vi "Load-deposition-file.vi"(8 "error in (no error)":errorcluster, 11 "Object ref in":T1) -> (0 "error out":errorcluster, 1 "Succes?":bool, 3 "Object ref out":T1)   [LabVIEW 2013, in "SLMControl.lvlib" / "SC-Main.lvclass"]
uses:
  SC-Main.lvclass
  Object-reference.ctl
  Client/Sources/Supported-modules.ctl
  SC-Main.lvclass/SC-Main.ctl
  Read Deposition status.vi
  Read Deposition file index.vi
  Read Deposition files.vi
  Read Client.vi
  Client/Sources/SC-Client.lvclass
  SA-SLMAPI/Sources/Load-file/Load-file.lvclass
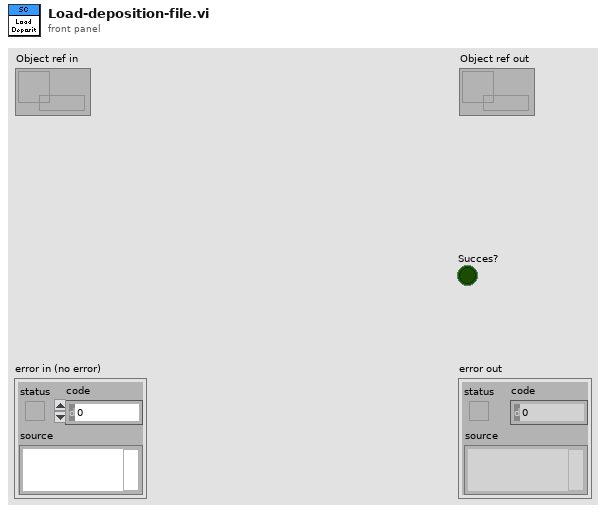
[diagram p1: front panel]
types:
  T1 = typedef "SLMControl.lvlib/SC-Main.lvclass/Object-reference.ctl" = refnum<data-value>
  T2 = typedef "SLMControl.lvlib/SC-Client.lvclass/Supported-modules.ctl" = enum16{"Server", "All", "SLMControl", "PowderDeposition", "StrategyParser", "CameraVision", "MaterialCharacterization", "StatusMonitor", "SLMSimulation", "LaserCharacterization"}
  T3 = typedef "SLMControl.lvlib/SC-Client.lvclass/Object-reference.ctl" = refnum<data-value>
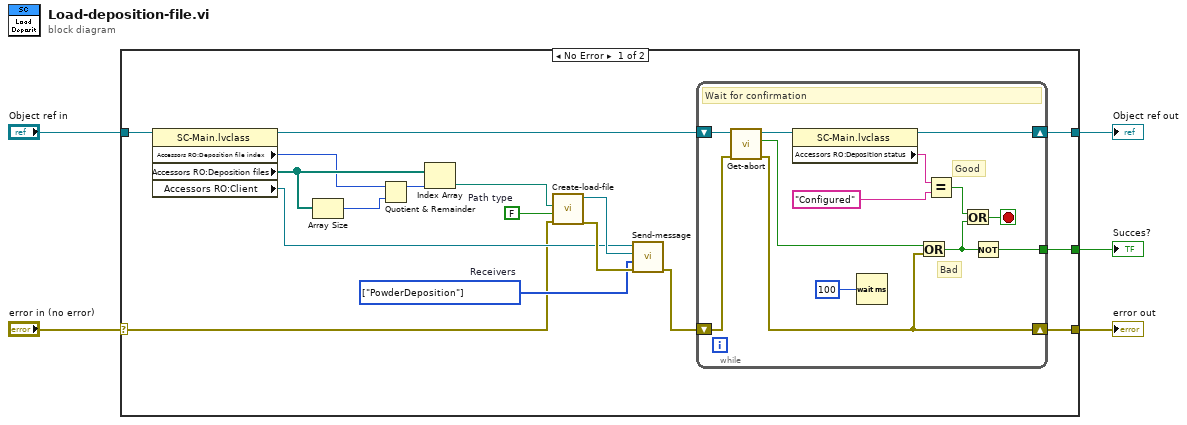
[diagram p0: block diagram]
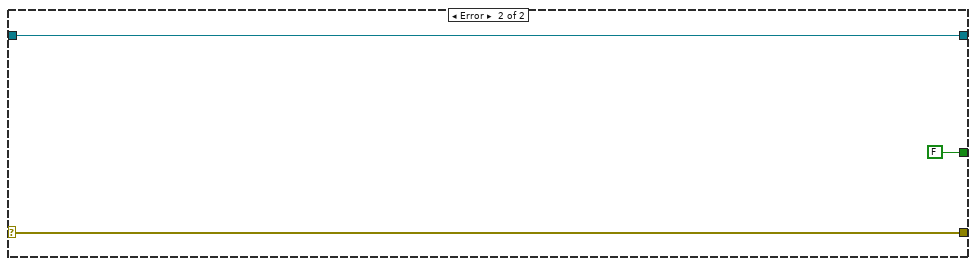
[diagram p2: hidden frame]
diagram:
  n1 = case shown="No Error" "error in (no error)" {
    selector: "error in (no error)" -> [w12 w38]
    tunnel: [w11 w38] -> w4
    tunnel: [w9 w37] -> w2
    tunnel: "Object ref in" -> [w22 w37]
    tunnel: [w7 FALSE] -> w1
    frame No Error {
      w13 = T2[] [enum."PowderDeposition"] items=["Server", "All", "SLMControl", "PowderDeposition", "StrategyParser", "CameraVision", "MaterialCharacterization", "StatusMonitor", "SLMSimulation", "LaserCharacterization"]  # Receivers
      w18 = FALSE  # Path type
      n2 = property class="SC-Main.lvclass"(reference=w22) -> (reference out=w8:T1, "Accessors RO:Deposition file index"=w6:i32, "Accessors RO:Deposition files"=w19:path[], "Accessors RO:Client"=w15:T3)  [unwired: 1 in, 1 out]
      n3 = Array Size(array=w19) -> (size(s)=w20:i32)
      n4 = Quotient & Remainder(x=w6, y=w20) -> (x-y*floor(x/y)=w21:i32)  [unwired: 1 out]
      n5 = Index Array(array=w19, index=w21) -> (element=w14:path)
      n6 = call "Create-load-file.vi"("error in (no error)"=w12, "Path type"=w18, "File path"=w14) -> ("error out"=w16:errorcluster, "Load-file out"=w17:refnum<class "Load-file.lvclass">)  [unwired: 7 in]
      n7 = call "Send-message.vi"("error in (no error)"=w16, "Receivers"=w13, "Message"=w17, "Client in"=w15) -> ("error out"=w10:errorcluster)  [unwired: 6 in, 1 out]
      n8 = while {
        shift-right: [w24] -> w11
        shift-left: w10 -> [w32]
        shift-right: [w34] -> w9
        shift-left: w8 -> [w35]
        tunnel: [w25] -> w7
        stop <- w29 stop-if-true
        # "Bad"
        # "Good"
        # "Wait for confirmation"
        n9 = call "Get-abort.vi"("error in (no error)"=w32, "Object ref in"=w35) -> ("error out"=w24:errorcluster, "Abort"=w26:bool, "Object ref out"=w33:T1)  [unwired: 7 in]
        n10 = property class="SC-Main.lvclass"(reference=w33) -> (reference out=w34:T1, "Accessors RO:Deposition status"=w31:string)  [unwired: 1 in, 1 out]
        n11 = Wait (ms)(milliseconds to wait=u32 100) -> ()  [unwired: 1 out]
        n12 = Or(x=w26, y=w24) -> (x .or. y?=w23:bool)
        n13 = Equal?(x=w31, y="Configured") -> (x = y?=w28:bool)
        n14 = Or(x=w28, y=w23) -> (x .or. y?=w29:bool)
        n15 = Not(x=w23) -> (.not. x?=w25:bool)
      }
    }
    frame Error {
    }
  }
  "error out" <- w4
  "Object ref out" <- w2
  "Succes?" <- w1
